vi "FlattenPages.vi"(10 "3D array in":dbl[][][](array[numeric])) -> (2 "2D array out":dbl[][](array[numeric]))   [LabVIEW 2022 SP3]
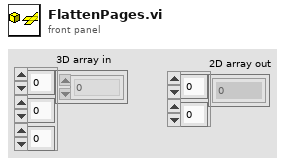
[diagram p1: front panel]
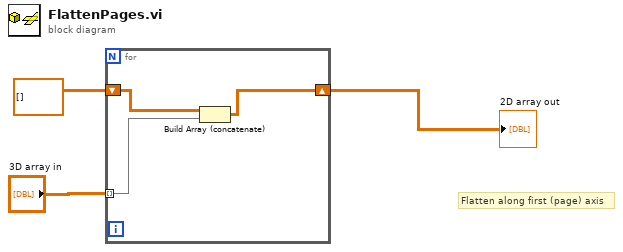
[diagram p0: block diagram]
diagram:
  # "Flatten along first (page) axis"
  n1 = for {
    tunnel: "3D array in" -> [w5] mode=indexing
    shift-right: [w6] -> w2
    shift-left: dbl[][] [] -> [w4]
    n2 = Build Array (concatenate)(w4, w5) -> (w6:dbl[][])
  }
  "2D array out" <- w2
